vi "Set-control-enable-single.vi"(8 "error in (no error)":errorcluster, 9 "Enable?":bool, 10 "Control name":T1, 11 "UI ref. in":refnum<data-value>) -> (0 "error out":errorcluster, 3 "UI ref.":refnum<data-value>)   [LabVIEW 2013, in "CameraVision.lvlib" / "CV-UI.lvclass"]
uses:
  CV-UI.lvclass
  Control-names.ctl
  CV-UI.lvclass/CV-UI.ctl
  Read Control refs.vi
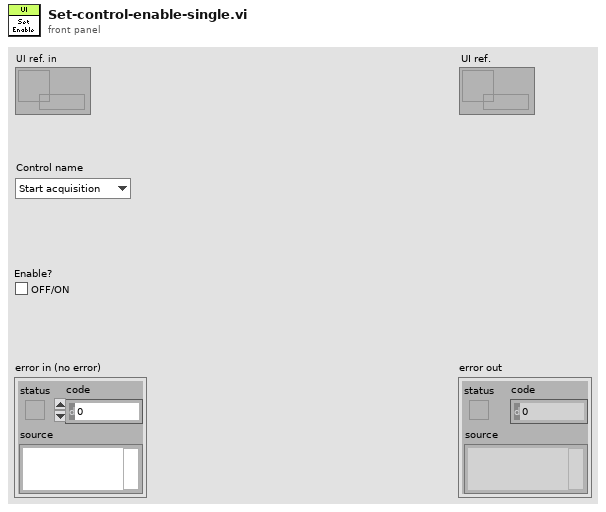
[diagram p1: front panel]
types:
  T1 = typedef "CameraVision.lvlib/CV-UI.lvclass/Control-names.ctl" = enum16{"Start acquisition", "Activate", "Stop acquisition", "Settings type", "Load settings", "Save settings", "Import images", "Camera selector", "Image type selector", "Batch browser", "Image refresh", "Parameter tabs", "Displays", "Processing tabs", "Processing selector", "Map characteristic", "Show info", "Manual trigger"}
  T2 = enum8{"Enabled", "Disabled", "Disabled and Grayed Out"}
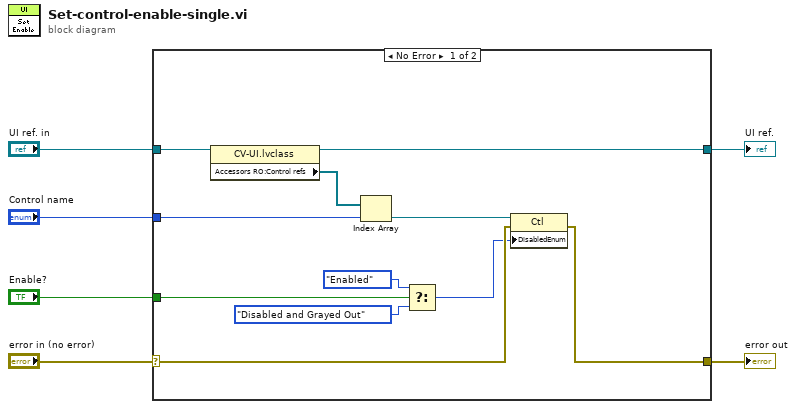
[diagram p0: block diagram]
diagram:
  n1 = case shown="No Error" "error in (no error)" {
    selector: "error in (no error)" -> [w11 w18]
    tunnel: [w14 w18] -> w5
    tunnel: [w13 w19] -> w3
    tunnel: "UI ref. in" -> [w17 w19]
    tunnel: "Control name" -> [w15 _]
    tunnel: "Enable?" -> [w10 _]
    frame No Error {
      n2 = property class="CV-UI.lvclass"(reference=w17) -> (reference out=w13:refnum<data-value>, "Accessors RO:Control refs"=w16:refnum<vi>[])  [unwired: 1 in, 1 out]
      n3 = Index Array(array=w16, index=w15) -> (element=w12:refnum<vi>)
      n4 = Select(t=T2."Enabled" ("Disabled"), s=w10, f=T2."Disabled and Grayed Out" ("Disabled")) -> (s? t:f=w9:T2)
      n5 = property class="Ctl"(reference=w12, error in=w11, "DisabledEnum"=w9) -> (error out=w14:errorcluster)  [unwired: 1 out]
    }
    frame Error {
    }
  }
  "error out" <- w5
  "UI ref." <- w3
